vi "Camera Manager Set Camera Param.vi"(8 "error in (no error)":errorcluster, 9 "Value":string, 10 "NodeName":string, 11 "cameraId":i32) -> (0 "error out":errorcluster, 1 "Value out":string, 2 "NodeName out":string, 3 "function return":bool)   [LabVIEW 2017, in "PlayNitrideCameraComponet1010_4.lvlib"]
doc: "__declspec(dllexport) bool CameraManager_SetCameraParam(int cameraId, char* NodeName, char* Value);"
uses:
  <userlib>/PlayNitrideCameraComponet1010_4/PlayNitrideCameraComponet1010_4.lvlib
  <userlib>/PlayNitrideCameraComponet1010_4/PlayNitrideCameraComponet.dll
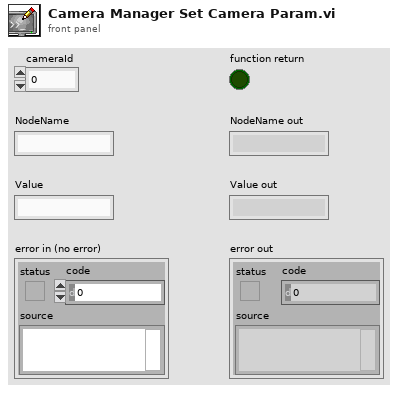
[diagram p1: front panel]
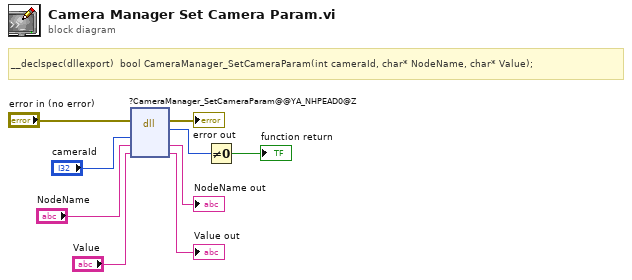
[diagram p0: block diagram]
diagram:
  # "__declspec(dllexport)  bool CameraManager_SetCameraParam(int cameraId, char* NodeName, char* Value);"
  n1 = dll-call lib="C:/Program Files/National Instruments/LabVIEW 2017/user.lib/PlayNitrideCameraComponet1010_4/PlayNitrideCameraComponet.*" fn="?CameraManager_SetCameraParam@@YA_NHPEAD0@Z"(error in="error in (no error)", "cameraId"="cameraId", "NodeName"="NodeName", "Value"="Value") -> (error out=→"error out":errorcluster, w8:u8, "NodeName"=→"NodeName out":string, "Value"=→"Value out":string)  [unwired: 3 in, 1 out]
  n2 = Not Equal To 0?(x=w8) -> (x != 0?=→"function return":bool)
